vi "Calibrate_Camera.vi"() -> ()   [LabVIEW 2017]
uses:
  <vilib>/userdefined/High Color/IMAQdx.ctl
  <vilib>/vision/driver/NI_Vision_Acquisition_Software.lvlib
panel:
  in  "stop":bool
  in  "Refnum in":T1="cam1"
  out "Image":T2(plugin-control)
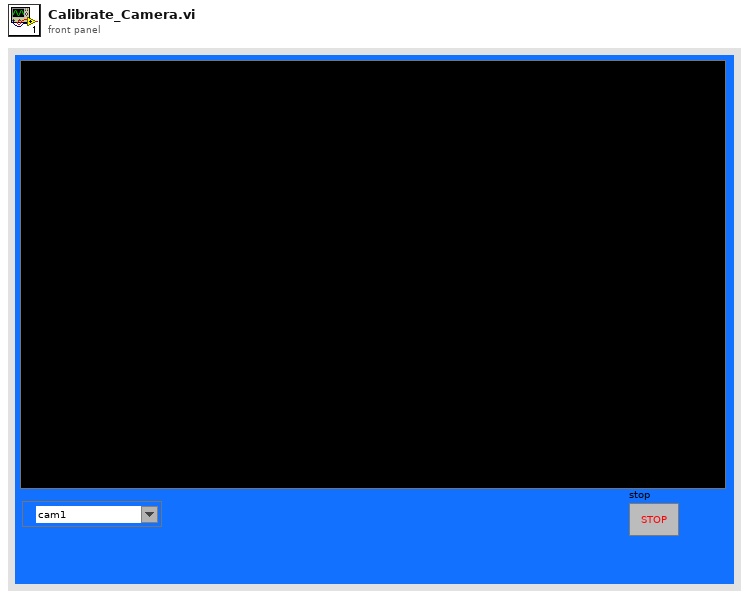
[diagram p1: front panel]
types:
  T1 = typedef "IMAQdx.ctl" = refnum<k21>
  T2 = typedef "IMAQ Image.ctl" = refnum<image>
  T3 = typedef "Image Type" = u32
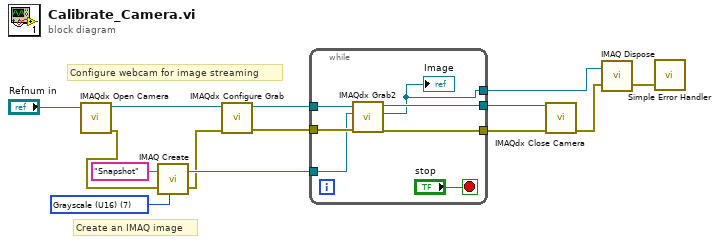
[diagram p0: block diagram]
diagram:
  w8 = T3 7 items=["Grayscale (U8)", "Grayscale (I16)", "Grayscale (SGL)", "Complex (CSG)", "RGB (U32)", "HSL (U32)", "RGB (U64)", "Grayscale (U16)"] ("Image Type")
  # "Create an IMAQ image"
  # "Configure webcam for image streaming"
  n1 = call <vilib>:"IMAQdx Open Camera.vi"("Session In"="Refnum in") -> ("error out"=w6:errorcluster, "Session Out"=w14:T1)  [unwired: 9 in]
  n2 = call "IMAQ Create"("Image Name"="Snapshot", "Image Type"=w8, "error in (no error)"=w6) -> ("New Image"=w7:T2, "error out"=w5:errorcluster)  [unwired: 2 in]
  n3 = call <vilib>:"IMAQdx Configure Grab.vi"("error in"=w5, "Session In"=w14) -> ("error out"=w12:errorcluster, "Session Out"=w13:T1)  [unwired: 8 in]
  n4 = while {
    tunnel: w13 -> [w21]
    tunnel: w12 -> [w20]
    tunnel: [w19] -> w10
    tunnel: [w18] -> w9
    tunnel: w7 -> [w16]
    tunnel: [w15] -> w3
    stop <- "stop" stop-if-true
    n5 = call <vilib>:"IMAQdx Grab2.vi"("error in"=w20, "Image In"=w16, "Session In"=w21) -> ("error out"=w19:errorcluster, "Image Out"=w15:T2, "Session Out"=w18:T1)  [unwired: 5 in, 1 out]
    "Image" <- w15
  }
  n6 = call <vilib>:"IMAQdx Close Camera.vi"("error in"=w10, "Session In"=w9) -> ("error out"=w2:errorcluster)  [unwired: 9 in]
  n7 = call "IMAQ Dispose"("Image"=w3, "error in (no error)"=w2) -> ("error out"=w1:errorcluster)  [unwired: 4 in]
  n8 = call <vilib>:"Simple Error Handler.vi"("error in (no error)"=w1) -> ()  [unwired: 4 in, 5 out]
